vi "Save_Time_Traces_low.vi"(0 "Data Type":T1, 1 "Full Header Info?":bool, 2 "Put each block into separate file":bool, 3 "Precision":i16=2, 5 "No of desired samples/ch":i32, 7 "Data to save":i32[](array[ring])=[1] items=["LDA (V)", "LDA (U)", "Save Nothing"], 9 "File Extension":string=".xls", 11 "Down Sample":i32=1, 12 "Leave space between blocks?":bool, 13 "Time Series":enum16{"Milliseconds", "Seconds"}(ring), 14 "Separation Character":string="\t") -> ()   [LabVIEW 2012]
uses:
  Controls/Instrument_Array.ctl
  Globals/Meas_global.vi
  Acquisition/PWA/PWAtasksGLOBAL.vi
  Globals/Plug_in_data_global.vi
  Globals/LDA_meas_global_1.vi
panel:
  # "Run this VI to update the channel names"
  # "0 means disabled"
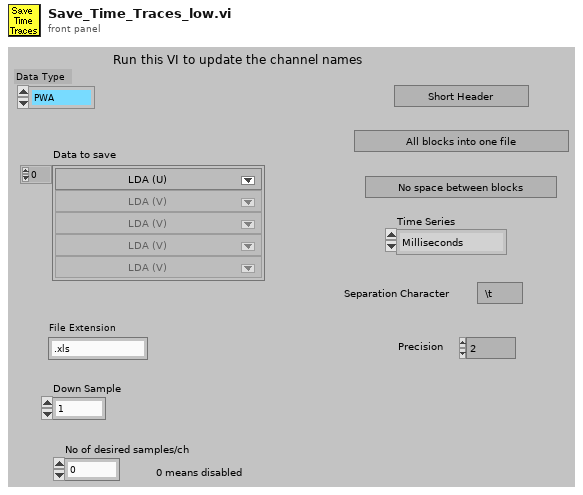
[diagram p1: front panel]
types:
  T1 = typedef "Instrument_Array.ctl" = enum16{"PWA", "LDA", "Analogue"}
  T2 = typedef "Analysis_info_cluster.ctl" = cluster{"Colour":u32, "Inst type":T3, "Inst name":string, "Symbol":string, "Code name":string, "Extra Info":string, "Inst Array":T1, "Extra Titles":string[], "Extra Values":string[], "U":dbl, "u^2":dbl, "u^3":dbl, "u^4":dbl, "Skew_u":dbl, "Kurt_u":dbl, "Sd Error in Mean":dbl, "% u'/U":dbl, "X":dbl, "Y":dbl, "Z":dbl, "Timescale integral to 25%":dbl, "Sd Error in Variance":dbl, "Calib File":path, "Calib Constants":dbl[], "Output Position":bool, "Full Stats":bool, "Av Sampling Rate":dbl, "Av No of Samples":dbl, "Total Meas Time (s)":dbl, "ADAM Ch Name":string}
  T3 = typedef "Inst_type.ctl" = enum16{"Propeller anemometer", "Raw voltage", "Pressure Transducer", "Pitot-static tube", "Preston tube", "Hot wire", "Cross wire 1", "Cross wire 2", "Generic Linear", "Generic Polynomial", "Generic BackPoly", "Fast FID", "Thermocouple", "Cold wire", "Pulsed Wire", "LDA Vel", "LDA Tran time", "LDA Arr time"}
  T4 = typedef "Time_Trace_Cluster.ctl" = cluster{"Weighting":dbl[], "Time (s)":dbl[], "Voltage":dbl[], "Eng Values":dbl[]}
  T5 = typedef "Trigger_Mode.ctl" = enum16{"Free Running", "Start on Trigger", "Trigger Every Block", "Trigger Every Sample"}
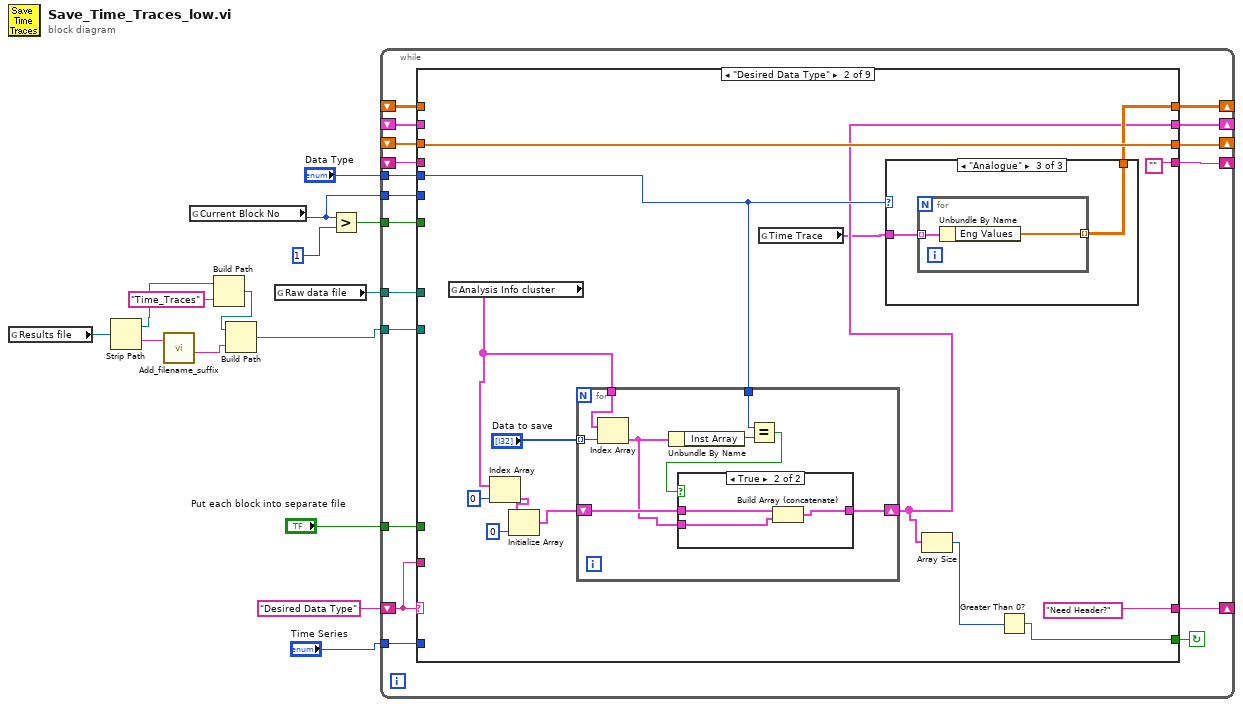
[diagram p0: block diagram]
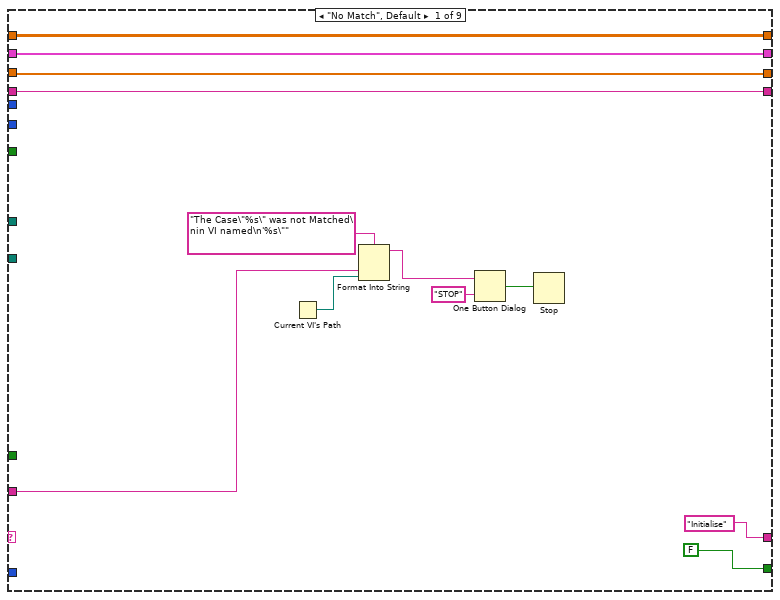
[diagram p2: hidden frame]
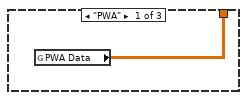
[diagram p4: hidden frame]
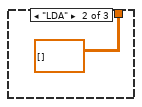
[diagram p5: hidden frame]
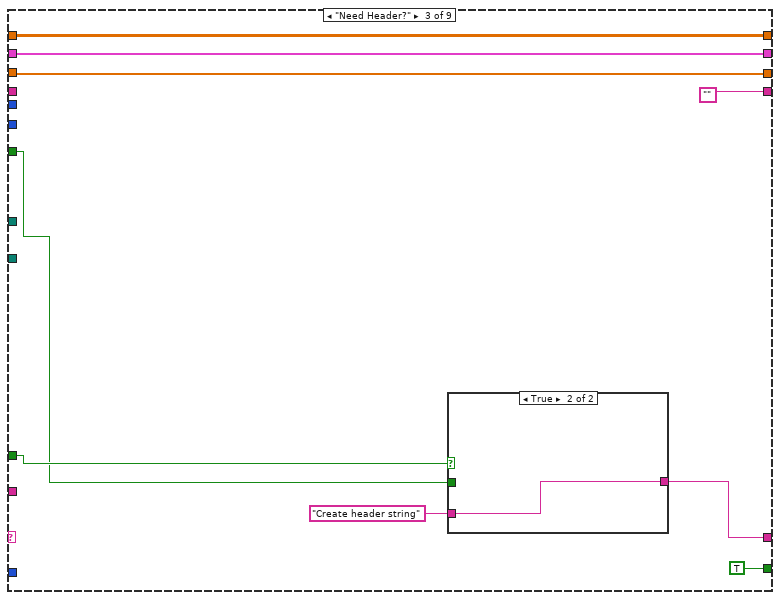
[diagram p6: hidden frame]
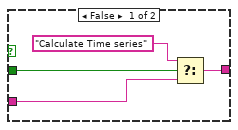
[diagram p7: hidden frame]
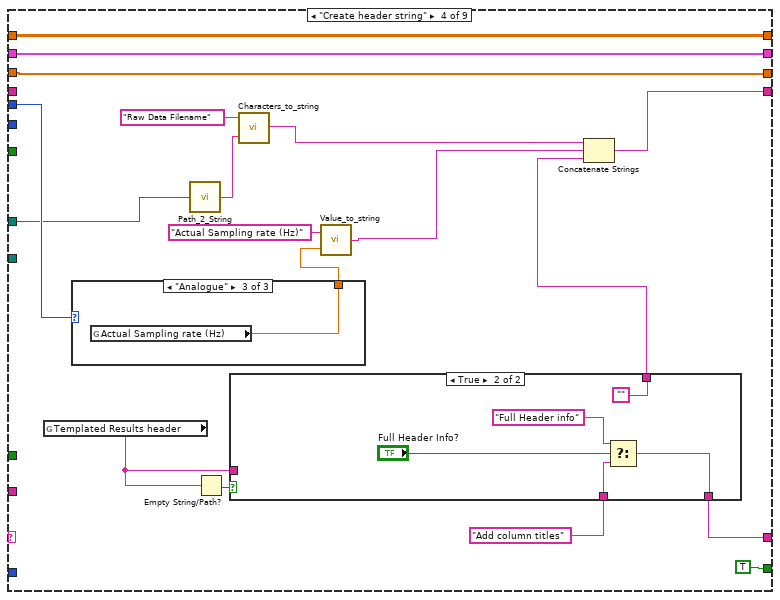
[diagram p8: hidden frame]
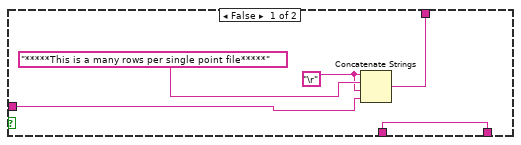
[diagram p9: hidden frame]
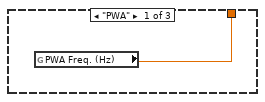
[diagram p10: hidden frame]
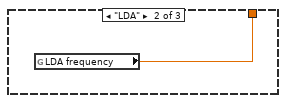
[diagram p11: hidden frame]
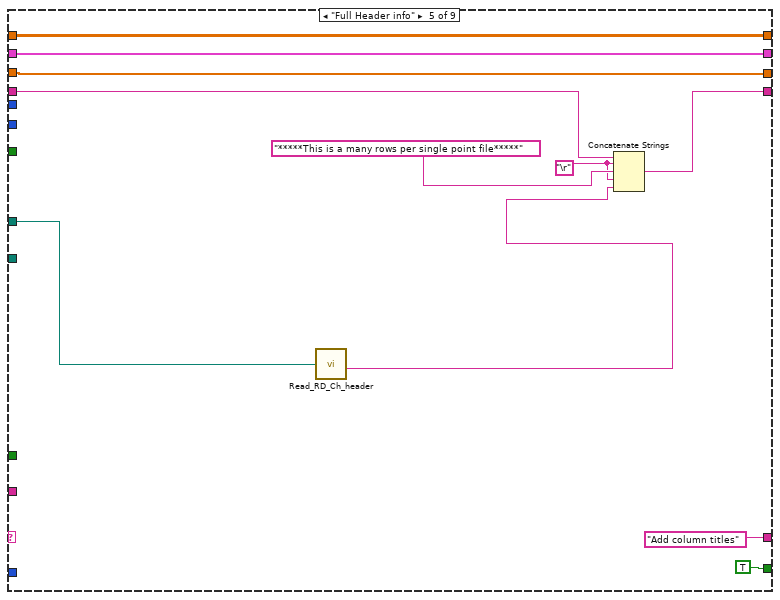
[diagram p12: hidden frame]
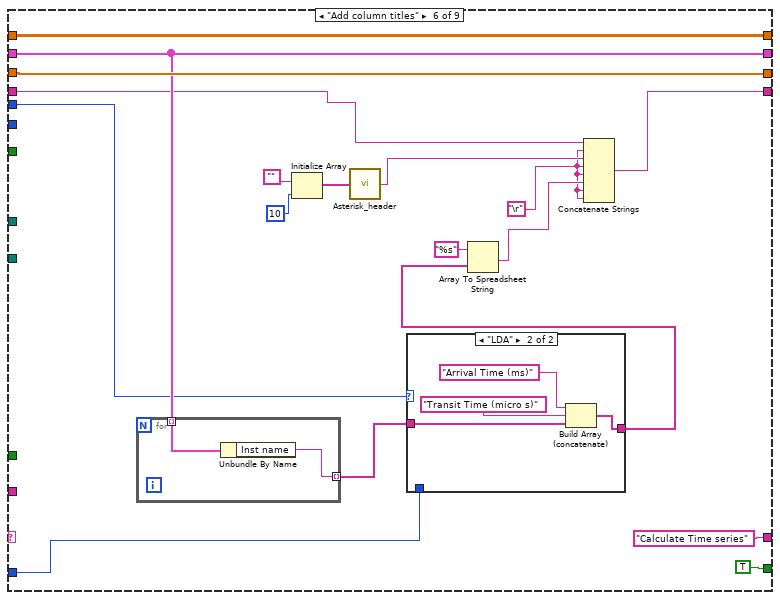
[diagram p13: hidden frame]
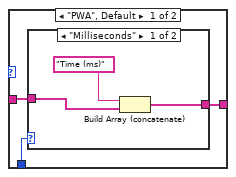
[diagram p14: hidden frame]
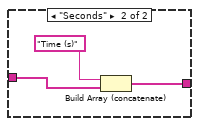
[diagram p15: hidden frame]
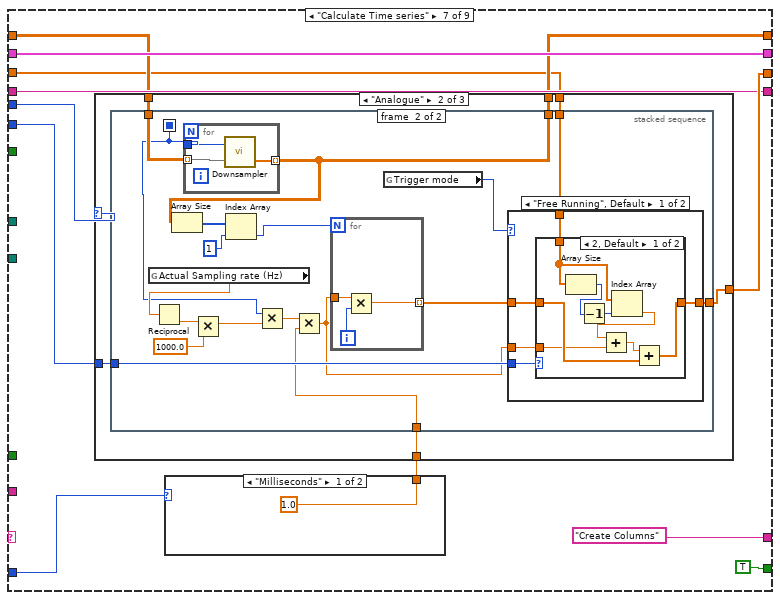
[diagram p16: hidden frame]
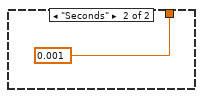
[diagram p17: hidden frame]
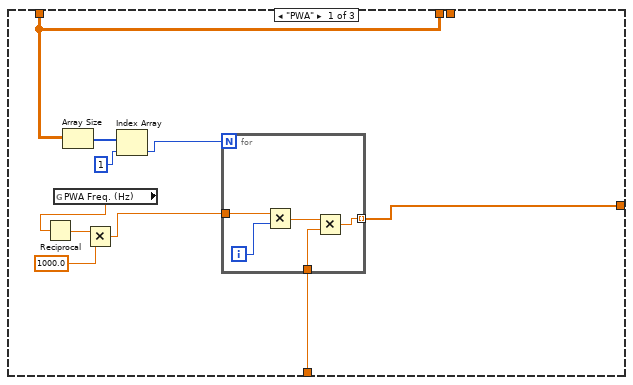
[diagram p18: hidden frame]
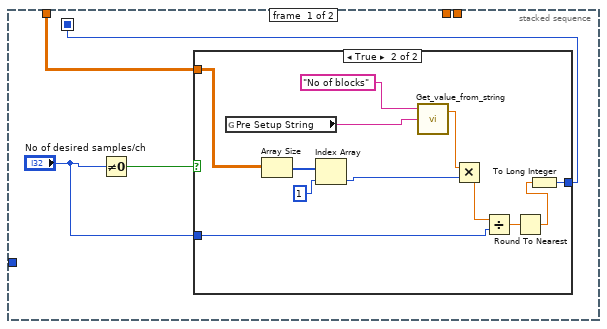
[diagram p19: hidden frame]
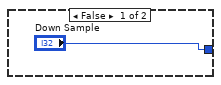
[diagram p20: hidden frame]
diagram:
  n1 = global read "Meas_global.vi" "Results file"() -> (w7:path)
  n2 = Strip Path(path=w7) -> (stripped path=w3:path, name=w6:string)
  n3 = call "Add_filename_suffix.vi"("Filename"=w6) -> ("Base name"=w5:string)  [unwired: 1 in, 3 out]
  n4 = global read "Meas_global.vi" "Current Block No"() -> (w11:i32)
  n5 = Build Path(base path=w3, name or relative path="Time_Traces") -> (appended path=w1:path)
  n6 = Build Path(base path=w1, name or relative path=w5) -> (appended path=w4:path)
  n7 = global read "Meas_global.vi" "Raw data file"() -> (w8:path)
  n8 = Greater?(x=w11, y=1) -> (0:w12:bool)
  n9 = while {
    shift-left: "Desired Data Type" -> [w31]
    shift-right: [w32] -> _
    shift-right: [w28] -> _
    shift-left: _ -> [w27]
    tunnel: "Put each block into separate file" -> [w30]
    tunnel: w8 -> [w29]
    tunnel: w12 -> [w26]
    shift-right: [w25] -> _
    shift-left: _ -> [w24]
    tunnel: w11 -> [w23]
    shift-right: [w22] -> _
    shift-left: _ -> [w21]
    tunnel: "Time Series" -> [w20]
    tunnel: "Data Type" -> [w19]
    shift-right: [w18] -> _
    shift-left: _ -> [w17]
    tunnel: w4 -> [w16]
    stop <- w33 continue-if-true
    n10 = case shown="\"Desired Data Type\"" w31 {
      tunnel: [FALSE w48 TRUE TRUE TRUE TRUE TRUE TRUE FALSE] -> w33
      tunnel: ["Initialise" "Need Header?" w84 w94 "Add column titles" ("t") "Calculate Time series" ("t") "Create Columns" ("t") "Write File" "End" ("t")] -> w32
      tunnel: w31 -> [w40 _ _ _ _ _ _ _ _]
      tunnel: w30 -> [_ _ w83 _ _ _ _ _ w348]
      tunnel: w29 -> [_ _ _ w99 w125 _ _ _ w358]
      tunnel: [w37 "" "" w107 w126 w150 w176 w277 w354] -> w28
      tunnel: w27 -> [w37 _ _ _ w127 w141 w176 w279 w354]
      tunnel: w26 -> [_ _ w82 _ _ _ _ _ w344]
      tunnel: [w36 w59 w86 w106 w133 w148 w178 w271 w351] -> w25
      tunnel: w24 -> [w36 w59 w86 w106 w133 w148 w169 w271 w351]
      tunnel: w23 -> [_ _ _ _ _ _ w168 _ w350]
      tunnel: [w35 w58 w79 w103 w132 w146 w170 w275 w345] -> w22
      tunnel: w21 -> [w35 _ w79 w103 w132 w146 w171 w275 w345]
      tunnel: w20 -> [_ _ _ _ _ w135 w175 w274 _]
      tunnel: w19 -> [_ w55 _ w101 _ w138 w173 w270 w340]
      tunnel: [w34 w47 w80 w100 w130 w145 w172 w272 w341] -> w18
      tunnel: w17 -> [w34 _ w80 w100 w130 w145 w172 w272 w341]
      tunnel: w16 -> [_ _ _ _ _ _ _ _ w337]
      frame "No Match", Default {
        n11 = Current VI's Path() -> (path=w39:path)
        n12 = Format Into String(format string="The Case\"%s\" was not Matched\nin VI named\n'%s\"" ("Format String"), w40, w39) -> (resulting string=w43:string)  [unwired: 2 in, 1 out]
        n13 = One Button Dialog(message=w43, button name ("OK")="STOP") -> (true=w41:bool)
        n14 = Stop(stop? (T)=w41) -> ()
      }
      frame "Desired Data Type" {
        n15 = global read "Meas_global.vi" "Analysis Info cluster"() -> (w51:T2[])
        n16 = Index Array(array=w51, index=0) -> (element=w52:T2)
        n17 = Initialize Array(w52, 0 ("dimension size")) -> (w54:T2[])
        n18 = for {
          tunnel: w51 -> [w68]
          tunnel: "Data to save" -> [w67] mode=indexing
          tunnel: w55 -> [w65]
          shift-right: [w61] -> w47
          shift-left: w54 -> [w63]
          n19 = Index Array(array=w68, index=w67) -> (element=w62:T2)
          n20 = Unbundle By Name(w62) -> ("Inst Array"=w66:T1)
          n21 = Equal?(x=w65, y=w66) -> (x = y?=w64:bool)
          n22 = case shown="True" w64 {
            tunnel: w63 -> [w69 w72]
            tunnel: w62 -> [_ w71]
            tunnel: [w69 w70] -> w61
            frame False {
            }
            frame True {
              n23 = Build Array (concatenate)(w72, w71) -> (w70:T2[])
            }
          }
        }
        n24 = global read "Meas_global.vi" "Time Trace"() -> (w46:T4[])
        n25 = case shown="\"Analogue\"" w55 {
          tunnel: [w73 dbl[][] [] ("Eng Values") w75] -> w58
          tunnel: w46 -> [_ _ w76]
          frame "PWA" {
            n26 = global read "PWAtasksGLOBAL.vi" "PWA Data"() -> (w73:dbl[][])
          }
          frame "LDA" {
          }
          frame "Analogue" {
            n27 = for {
              tunnel: w76 -> [w78] mode=indexing
              tunnel: [w77] -> w75 mode=indexing
              n28 = Unbundle By Name(w78) -> ("Eng Values"=w77:dbl[])
            }
          }
        }
        n29 = Array Size(array=w47) -> (size(s)=w49:i32)
        n30 = Greater Than 0?(x=w49) -> (x > 0?=w48:bool)
      }
      frame "Need Header?" {
        n31 = case shown="True" w83 {
          tunnel: [w91 w92] -> w84
          tunnel: w82 -> [w90 _]
          tunnel: "Create header string" -> [w88 w92]
          frame False {
            n32 = Select(t="Calculate Time series", s=w90, f=w88) -> (s? t:f=w91:string)
          }
          frame True {
          }
        }
      }
      frame "Create header string" {
        n33 = global read "Plug_in_data_global.vi" "Templated Results header"() -> (w96:string)
        n34 = case shown="\"Analogue\"" w101 {
          tunnel: [w121 w122 w123] -> w102
          frame "PWA" {
            n35 = global read "PWAtasksGLOBAL.vi" "PWA Freq. (Hz)"() -> (w121:dbl)
          }
          frame "LDA" {
            n36 = global read "Meas_global.vi" "LDA frequency"() -> (w122:dbl)
          }
          frame "Analogue" {
            n37 = global read "Meas_global.vi" "Actual Sampling rate (Hz)"() -> (w123:dbl)
          }
        }
        n38 = call "Path_2_String.vi"("Real Path"=w99) -> ("Path String"=w98:string)
        n39 = Empty String/Path?(string/path=w96) -> (empty?=w97:bool)
        n40 = case shown="True" w97 {
          tunnel: w96 -> [w113 _]
          tunnel: "Add column titles" ("t") -> [w112 w118]
          tunnel: [w112 w117] -> w94
          tunnel: [w111 ""] -> w93
          frame False {
            w114 = "\r"
            n41 = Concatenate Strings(w114, "*****This is a many rows per single point file*****", w114, w113) -> (w111:string)
          }
          frame True {
            n42 = Select(t="Full Header info", s="Full Header Info?", f=w118) -> (s? t:f=w117:string)
          }
        }
        n43 = call "Characters_to_string.vi"("Characters to write"=w98, "Label for characters"="Raw Data Filename") -> ("Output string"=w109:string)
        n44 = call "Value_to_string.vi"("Value"=w102, "Label for value"="Actual Sampling rate (Hz)") -> ("Output string"=w104:string)  [unwired: 1 in]
        n45 = Concatenate Strings(w109, w104, w93) -> (w107:string)
      }
      frame "Full Header info" {
        w128 = "\r"
        n46 = call "Read_RD_Ch_header.vi"("Raw data file"=w125) -> ("Ch string"=w124:string)  [unwired: 3 out]
        n47 = Concatenate Strings(w127, w128, "*****This is a many rows per single point file*****", w128, w124) -> (w126:string)
      }
      frame "Add column titles" {
        w139 = "\r"
        n48 = for {
          tunnel: [w166] -> w137 mode=indexing
          tunnel: w145 -> [w167] mode=indexing
          n49 = Unbundle By Name(w167) -> ("Inst name"=w166:string)
        }
        n50 = Initialize Array("", 10) -> (w142:string[])
        n51 = call "Asterisk_header.vi"("Channel names"=w142) -> ("Header string"=w140:string)
        n52 = case shown="\"LDA\"" w138 {
          tunnel: w137 -> [w155 w163]
          tunnel: [w154 w162] -> w136
          tunnel: w135 -> [w153 _]
          frame "PWA", Default {
            n53 = case shown="\"Milliseconds\"" w153 {
              tunnel: w155 -> [w158 w161]
              tunnel: [w157 w160] -> w154
              frame "Milliseconds" {
                n54 = Build Array (concatenate)("Time (ms)", w158) -> (w157:string[])
              }
              frame "Seconds" {
                n55 = Build Array (concatenate)("Time (s)", w161) -> (w160:string[])
              }
            }
          }
          frame "LDA" {
            n56 = Build Array (concatenate)("Arrival Time (ms)", "Transit Time (micro s)", w163) -> (w162:string[])
          }
        }
        n57 = Array To Spreadsheet String(array=w136, 3:"%s" ("format string")) -> (spreadsheet string=w147:string)  [unwired: 1 out]
        n58 = Concatenate Strings(w141, w139, w140, w139, w139, w147, w139, w139) -> (w150:string)
      }
      frame "Calculate Time series" {
        n59 = case shown="\"Milliseconds\"" w175 {
          tunnel: [1.0 0.001] -> w174
          frame "Milliseconds" {
          }
          frame "Seconds" {
          }
        }
        n60 = case shown="\"Analogue\"" w173 {
          tunnel: [w183 w199 w260] -> w178
          tunnel: w174 -> [w185 w202 w261]
          tunnel: w171 -> [w182 w201 w259]
          tunnel: [w182 w200 w259] -> w170
          tunnel: w169 -> [_ w198 _]
          tunnel: w168 -> [_ w197 _]
          frame "PWA" {
            n61 = global read "PWAtasksGLOBAL.vi" "PWA Freq. (Hz)"() -> (w184:dbl)
            n62 = Reciprocal(x=w184) -> (1/x=w191:dbl)
            n63 = Array Size(array=w182) -> (size(s)=w188:i32[])
            n64 = Multiply(x=w191, y=1000.0) -> (x*y=w189:dbl)
            n65 = Index Array(array=w188, index=1) -> (element=w186:i32)
            n66 = for {
              N: w186 -> [_]
              tunnel: w189 -> [w195]
              tunnel: [w193] -> w183 mode=indexing
              tunnel: w185 -> [w192]
              i -> [w196]
              n67 = Multiply(x=w195, y=w196) -> (x*y=w194:dbl)
              n68 = Multiply(x=w194, y=w192) -> (x*y=w193:dbl)
            }
          }
          frame "Analogue" {
            n69 = stacked-sequence {
              seq-local: [w204 _] -> [_ w224]
              tunnel: w202 -> [_ w221]
              tunnel: w201 -> [w206 w231]
              tunnel: [_ w229] -> w200
              tunnel: [_ w227] -> w199
              tunnel: w198 -> [_ w225]
              tunnel: w197 -> [_ w223]
              frame #0 {
                n70 = Not Equal To 0?(x="No of desired samples/ch") -> (x != 0?=w203:bool)
                n71 = case shown="True" w203 {
                  tunnel: w206 -> [_ w215]
                  tunnel: "No of desired samples/ch" -> [_ w211]
                  tunnel: ["Down Sample" w208] -> w204
                  frame False {
                  }
                  frame True {
                    n72 = global read "Meas_global.vi" "Pre Setup String"() -> (w218:string)
                    n73 = Array Size(array=w215) -> (size(s)=w217:i32[])
                    n74 = Index Array(array=w217, index=1) -> (element=w213:i32)
                    n75 = call "Get_value_from_string.vi"("Input string"=w218, "Variable name"="No of blocks") -> ("Value"=w214:dbl)  [unwired: 1 in, 1 out]
                    n76 = Multiply(x=w214, y=w213) -> (x*y=w212:dbl)
                    n77 = Divide(x=w212, y=w211) -> (x/y=w210:dbl)
                    n78 = Round To Nearest(number=w210) -> (nearest integer value=w209:dbl)
                    n79 = To Long Integer(number=w209) -> (32bit integer=w208:i32)
                  }
                }
              }
              frame #1 {
                n80 = global read "Meas_global.vi" "Actual Sampling rate (Hz)"() -> (w232:dbl)
                n81 = Reciprocal(x=w232) -> (1/x=w237:dbl)
                n82 = for {
                  tunnel: w231 -> [w255] mode=indexing
                  tunnel: w224 -> [w254]
                  tunnel: [w253] -> w229 mode=indexing
                  n83 = call "Downsampler.vi"("Input Array"=w255, "Averaging samples"=w254) -> ("Downsampled Array"=w253:dbl[])  [unwired: 1 out]
                }
                n84 = Array Size(array=w229) -> (size(s)=w235:i32[])
                n85 = Multiply(x=w237, y=1000.0) -> (x*y=w230:dbl)
                n86 = Index Array(array=w235, index=1) -> (element=w233:i32)
                n87 = Multiply(x=w224, y=w230) -> (x*y=w222:dbl)
                n88 = Multiply(x=w222, y=w221) -> (x*y=w220:dbl)
                n89 = for {
                  N: w233 -> [_]
                  tunnel: w220 -> [w257]
                  tunnel: [w256] -> w226 mode=indexing
                  i -> [w258]
                  n90 = Multiply(x=w257, y=w258) -> (x*y=w256:dbl)
                }
                n91 = global read "Meas_global.vi" "Trigger mode"() -> (w228:T5)
                n92 = case shown="\"Free Running\", Default" w228 {
                  tunnel: w223 -> [w242 _]
                  tunnel: [w241 w252] -> w227
                  tunnel: w226 -> [w240 w252]
                  tunnel: w225 -> [w239 _]
                  tunnel: w220 -> [w238 _]
                  frame "Free Running", Default {
                    n93 = case shown="2, Default" w242 {
                      tunnel: [w246 w251] -> w241
                      tunnel: w240 -> [w247 w251]
                      tunnel: w239 -> [w248 _]
                      tunnel: w238 -> [w243 _]
                      frame 2, Default {
                        n94 = Array Size(array=w248) -> (size(s)=w249:i32)
                        n95 = Decrement(x=w249) -> (x-1=w250:i32)
                        n96 = Index Array(array=w248, index=w250) -> (element=w244:dbl)
                        n97 = Add(x=w244, y=w243) -> (x+y=w245:dbl)
                        n98 = Add(x=w245, y=w247) -> (x+y=w246:dbl[])
                      }
                      frame 1 {
                      }
                    }
                  }
                  frame "Trigger Every Block" {
                  }
                }
              }
            }
          }
          frame "LDA" {
            n99 = global read "LDA_meas_global_1.vi" "Arrival times"() -> (w263:dbl[])
            n100 = for {
              shift-right: [w266] -> _
              shift-left: 0.0 -> [w268]
              tunnel: w263 -> [w267] mode=indexing
              tunnel: [w265] -> w260 mode=indexing
              tunnel: w261 -> [w264]
              n101 = Add(x=w268, y=w267) -> (x+y=w266:dbl)
              n102 = Multiply(x=w266, y=w264) -> (x*y=w265:dbl)
            }
          }
        }
      }
      frame "Create Columns" {
        n103 = Array Size(array=w272) -> (size(s)=w282:i32)
        n104 = Decrement(x=w282) -> (x-1=w283:i32)
        n105 = global read "LDA_meas_global_1.vi" "Transit times"() -> (w269:dbl[])
        n106 = for {
          shift-right: [w300] -> w278
          shift-left: "" -> [w295]
          tunnel: "Separation Character" -> [w286]
          tunnel: w272 -> [w290]
          tunnel: w275 -> [w298]
          tunnel: w283 -> [w294]
          tunnel: w271 -> [w292] mode=indexing
          tunnel: w274 -> [w291]
          tunnel: w270 -> [w289]
          tunnel: w269 -> [w288]
          i -> [w287]
          n107 = case shown="\"Milliseconds\"" w291 {
            tunnel: [w312 w316] -> w285
            tunnel: w286 -> [w311 w315]
            tunnel: w292 -> [w310 w314]
            frame "Seconds" {
              n108 = Format Into String(format string="%.4f%s", w310, w311) -> (resulting string=w312:string)  [unwired: 2 in, 1 out]
            }
            frame "Milliseconds" {
              n109 = Format Into String(format string="%.2f%s", w314, w315) -> (resulting string=w316:string)  [unwired: 2 in, 1 out]
            }
          }
          n110 = Index Array(array=w298, index (col)=w287) -> (element=w297:dbl[])  [unwired: 1 in]
          n111 = case shown="\"PWA\", Default" w289 {
            tunnel: w288 -> [_ w308]
            tunnel: w287 -> [_ w307]
            tunnel: w286 -> [_ w304]
            tunnel: [w301 w303] -> w284
            tunnel: w285 -> [w301 w302]
            frame "PWA", Default {
            }
            frame "LDA" {
              n112 = Index Array(array=w308, index=w307) -> (element=w305:dbl)
              n113 = Format Into String(format string="%.2f%s", initial string=w302, w305, w304) -> (resulting string=w303:string)  [unwired: 1 in, 1 out]
            }
          }
          n114 = for {
            shift-right: [w324] -> w296
            shift-left: w284 -> [w326]
            tunnel: w286 -> [w323]
            tunnel: w297 -> [w319]
            tunnel: w294 -> [w322]
            tunnel: "Precision" -> [w320]
            tunnel: w290 -> [_] mode=indexing
            i -> [w318]
            n115 = Index Array(array=w319, index=w318) -> (element=w317:dbl)
            n116 = Equal?(x=w318, y=w322) -> (x = y?=w321:bool)
            n117 = Number To Fractional String(number=w317, precision (6)=w320) -> (F-format string=w325:string)  [unwired: 2 out]
            n118 = case shown="False" w321 {
              tunnel: w326 -> [w330 w333]
              tunnel: w325 -> [w329 w332]
              tunnel: [w328 w331] -> w324
              tunnel: w323 -> [w327 _]
              frame False {
                n119 = Concatenate Strings(w330, w329, w327) -> (w328:string)
              }
              frame True {
                n120 = Concatenate Strings(w333, w332) -> (w331:string)
              }
            }
          }
          n121 = Concatenate Strings(w295, w296, "\r") -> (w300:string)
        }
        n122 = Concatenate Strings(w279, w278) -> (w277:string)
      }
      frame "Write File" {
        n123 = Strip Path(path=w358) -> (name=w342:string)  [unwired: 1 out]
        n124 = call "Add_filename_suffix.vi"("Filename"=w342) -> ("Base name"=w343:string)  [unwired: 1 in, 3 out]
        n125 = case shown="\"LDA\"" w340 {
          tunnel: ["PWA" "AN" "LDA"] -> w339
          frame "PWA" {
          }
          frame "Analogue" {
          }
          frame "LDA" {
          }
        }
        n126 = case shown="False" w348 {
          tunnel: w343 -> [w364 w375]
          tunnel: w350 -> [_ w372]
          tunnel: [w363 w378] -> w349
          tunnel: w344 -> [w369 _]
          tunnel: [w369 FALSE] -> w347
          tunnel: [w368 w374] -> w346
          tunnel: w337 -> [w368 w376]
          tunnel: [2 ("y") 3 ("y")] -> _
          tunnel: w339 -> [w365 w371]
          tunnel: "File Extension" -> [w362 w370]
          frame False {
            n127 = Format Into String(format string="_%s%s", initial string=w364, w365, w362) -> (resulting string=w363:string)  [unwired: 1 in, 1 out]
          }
          frame True {
            n128 = Format Into String(format string="_%s_%d%s", initial string=w375, w371, w372, w370) -> (resulting string=w378:string)  [unwired: 1 in, 1 out]
            n129 = Build Path(base path=w376, name or relative path=w375) -> (appended path=w374:path)
          }
        }
        n130 = global read "Meas_global.vi" "Iteration Number"() -> (w335:i32)
        n131 = Build Path(base path=w346, name or relative path=w349) -> (appended path=w336:path)
        n132 = Equal To 0?(x=w335) -> (x = 0?=w334:bool)
        n133 = case shown="False" w347 {
          tunnel: [w380 w388] -> w356
          tunnel: w354 -> [w380 w387]
          tunnel: [w383 w386] -> w357
          tunnel: w336 -> [w382 w384]
          tunnel: [w381 w384] -> w355
          frame False {
            w383 = FALSE  # append to file? (new file:F)
            n134 = call "Create_directory_path.vi"("Path name"=w382) -> ("Path name Out"=w381:path)  [unwired: 1 in, 1 out]
          }
          frame True {
            w386 = TRUE  # append to file? (new file:F)
            n135 = case shown="True" "Leave space between blocks?" {
              tunnel: [w389 w392] -> w388
              tunnel: w387 -> [w389 w391]
              frame False {
              }
              frame True {
                n136 = Concatenate Strings("\r", w391) -> (w392:string)
              }
            }
          }
        }
        n137 = call "Write_Characters_To_File.vi"("file path (dialog if empty)"=w355, "advisory dialog? (display:T)"=w334, "character string"=w356, "append to file? (new file:F)"=w357) -> ()  [unwired: 1 in, 4 out]
      }
    }
  }
